vi "LoadCell.vi"(1 "tara":dbl, 2 "factor":dbl, 3 "data":dbl) -> (0 "force (Kgf)":dbl)   [LabVIEW 2014]
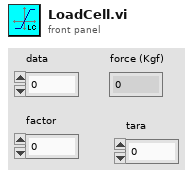
[diagram p1: front panel]
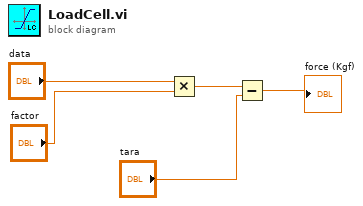
[diagram p0: block diagram]
diagram:
  n1 = Multiply(x="data", y="factor") -> (x*y=w3:dbl)
  n2 = Subtract(x=w3, y="tara") -> (x-y=→"force (Kgf)":dbl)
